vi "niRFUtil RFHS Math Divide and Assign Array by Array CSG.vi"(0 "data in":csg[](array[numeric]), 2 "RFHS?":bool=TRUE, 5 "divisor in":csg[](array[numeric]), 11 "error in":errorcluster) -> (4 "result out":csg[](array[numeric]), 15 "error out":errorcluster)   [LabVIEW 2015, in "niRFUtil.lvlib"]
uses:
  niRFUtil.lvlib
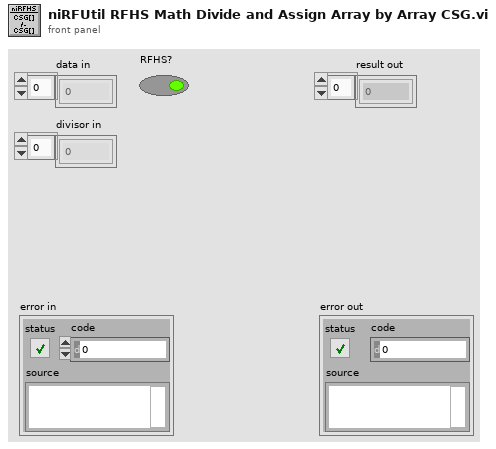
[diagram p1: front panel]
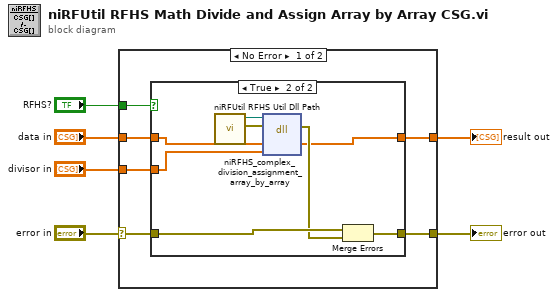
[diagram p0: block diagram]
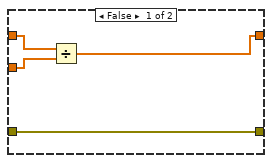
[diagram p2: hidden frame]
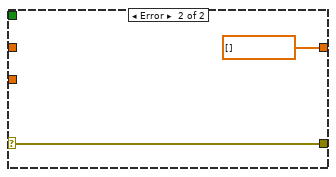
[diagram p3: hidden frame]
diagram:
  n1 = case shown="No Error" "error in" {
    selector: "error in" -> [w8 w26]
    tunnel: "RFHS?" -> [w12 _]
    tunnel: "data in" -> [w11 _]
    tunnel: "divisor in" -> [w10 _]
    tunnel: [w9 csg[] [] ("result")] -> w3
    tunnel: [w7 w26] -> w1
    frame No Error {
      n2 = case shown="True" w12 {
        tunnel: w11 -> [w16 w24]
        tunnel: w10 -> [w15 w23]
        tunnel: [w14 w17] -> w9
        tunnel: w8 -> [w13 w20]
        tunnel: [w13 w18] -> w7
        frame False {
          n3 = Divide(x=w16, y=w15) -> (x/y=w14:csg[])
        }
        frame True {
          n4 = call "niRFUtil RFHS Util Dll Path.vi"() -> ("error out"=w22:errorcluster, "Path"=w21:path)  [unwired: 7 in, 3 out]
          n5 = dll-call lib="R:/niRFHS.dll" fn="niRFHS_complex_division_assignment_array_by_array"(path in=w21, error in=w22, "data"=w24, "divisor"=w23) -> (error out=w19:errorcluster, "data"=w17:csg[])  [unwired: 3 in, 1 out]
          n6 = Merge Errors(w20, w19) -> (w18:errorcluster)
        }
      }
    }
    frame Error {
    }
  }
  "result out" <- w3
  "error out" <- w1
